vi "Force Arm Start.vi"(7 "Timeout (s)":dbl=10.0, 8 "Error In":errorcluster, 11 "ARM(T)/DISARM(F)":bool=TRUE) -> (0 "Error Out":errorcluster, 3 "Time out":bool)   [LabVIEW 2014]
uses:
  <vilib>/Platform/TimedLoop/XDataNode/timing_clust.ctl
  <vilib>/Platform/TimedLoop/XDataNode/nitl_modes.ctl
  <vilib>/Platform/TimedLoop/XDataNode/wakeup.ctl
  Aircraft Information/Sub VI/Get Aircraft Information.vi
  <vilib>/platform/TimedLoop/XDataNode/XDataNode.xnode
  <vilib>/Platform/TimedLoop/XDataNode/XDNodeRunTimeDep.lvlib
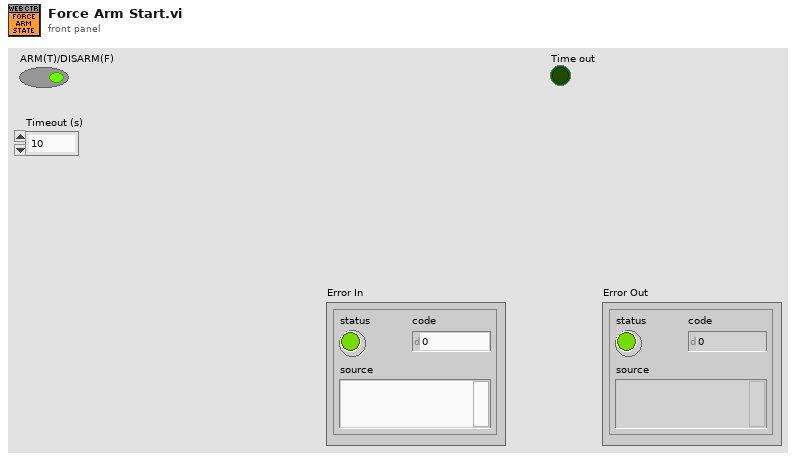
[diagram p1: front panel]
types:
  T1 = typedef "XDNodeRunTimeDep.lvlib/timing_clust.ctl" = cluster{"Expected End [f-1]":u64, "Actual End [f-1]":u64, "Finished Late? [f-1]":bool, "Expected End [i-1]":u64, "Actual End [i-1]":u64, "Finished Late? [i-1]":bool, "Expected Start [i]":u64, "Actual Start [i]":u64, "Expected Start [f]":u64, "Actual Start [f]":u64, "Source Name":string, "Structure Name":string, "Period":i64, "Deadline":i64, "Offset":i64, "Start":i64, "Priority":i32, "Timeout":i32, "Mode":T2, "Wakeup Reason":T3, "Error":errorcluster, "Source Type":string, "Secondary Source Type":string, "Global End Time":u64, "Global Start Time":u64, "Frame Duration":u64, "Iteration Duration":u64, "Assigned CPU":i32, "I/O Scan Engine Mode":u32}
  T2 = typedef "XDNodeRunTimeDep.lvlib/nitl_modes.ctl" = enum32{"No Change", "Process missed periods, maintain original phase", "Discard missed periods, maintain original phase", "Process missed periods, ignore original phase", "Discard missed periods, ignore original phase"}
  T3 = typedef "XDNodeRunTimeDep.lvlib/wakeup.ctl" = enum32{"Normal", "Aborted", "Asynchronous wakeup", "Timing source error", "Timed loop error", "Timeout"}
  T4 = typedef "Drone Information.ctl" = cluster{"Aircraft ID":u8, "Tag ID":string, "System Status":string, "Base Mode":T5, "Armed/Disarmed":bool, "Battery Voltage":dbl, "Control Mode":T6, "Initialisation":u8, "Coms with aircraft good":bool, "Mode":string, "Mission Uploaded":bool}
  T5 = typedef "Base Mode.ctl" = cluster{"Custom Mode":bool, "Test Enabled":bool, "Autonomous Mode":bool, "Guided Mode":bool, "Stabilization Enabled":bool, "HIL Enabled":bool, "Manual Mode":bool, "Arm":bool}
  T6 = typedef "Aircraft Mode.ctl" = enum16{"Loiter", "Stabalise", "Failsafe", "Emergency Stop"}
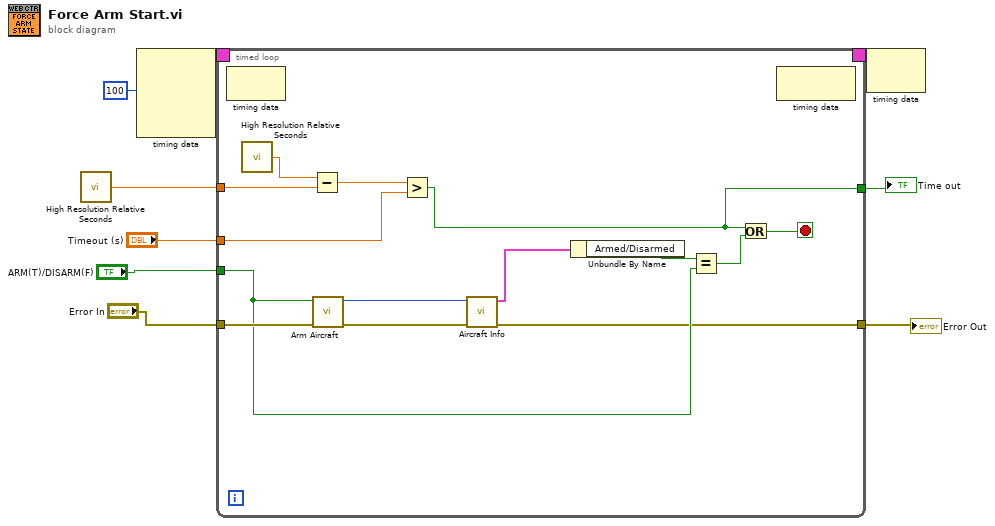
[diagram p0: block diagram]
diagram:
  n1 = call <vilib>:"High Resolution Relative Seconds.vi"() -> ("relative seconds"=w7:dbl)
  n2 = node-c288(i64 100 ("Period")) -> (w9:T1)  [unwired: 3 in]
  n3 = timed-loop {
    timing: w9 -> [_]
    timing-out: [_] -> w8
    tunnel: w7 -> [w22]
    tunnel: "Error In" -> [w15]
    tunnel: [w11] -> w4
    tunnel: "Timeout (s)" -> [w17]
    tunnel: "ARM(T)/DISARM(F)" -> [w12]
    tunnel: [w10] -> w1
    stop <- w16 stop-if-true
    n4 = node-c288() -> ()  [unwired: 1 in, 1 out]
    n5 = call <vilib>:"High Resolution Relative Seconds.vi"() -> ("relative seconds"=w23:dbl)
    n6 = Subtract(x=w23, y=w22) -> (x-y=w18:dbl)
    n7 = call "Arm Aircraft.vi"("Error In"=w15, "ARM(T)/DISARM(F)"=w12) -> ("error out"=w14:errorcluster, "Selected Aircraft ID Out"=w13:u8)  [unwired: 8 in]
    n8 = Greater?(x=w18, y=w17) -> (0:w10:bool)
    n9 = call-poly "Aircraft Info.vi"("Error In"=w14, "Aircraft ID"=w13) -> ("Error Out"=w11:errorcluster, "Aircraft Information Out"=w21:T4)  [unwired: 8 in]
    n10 = Unbundle By Name(w21) -> ("Armed/Disarmed"=w20:bool)
    n11 = Equal?(x=w20, y=w12) -> (x = y?=w19:bool)
    n12 = Or(x=w10, y=w19) -> (x .or. y?=w16:bool)
    n13 = node-c288() -> ()  [unwired: 1 in, 1 out]
  }
  "Error Out" <- w4
  "Time out" <- w1
  n14 = node-c288(w8) -> ()  [unwired: 1 out]
